vi "Fit to Decoration.vi"(8 "error in":errorcluster, 10 "Border":i32, 11 "Flex Subpanel in":refnum<class "Flex UI Subpanel.lvclass">) -> (0 "error out":errorcluster, 3 "Flex Subpanel out":refnum<class "Flex UI Subpanel.lvclass">)   [LabVIEW 2016, in "Flex UI Subpanel.lvclass"]
doc: "Resizes the subpanel around the largest decoration."
uses:
  Flex UI Subpanel.lvclass
  C:/VI Packages/Flex UI/Flex UI (Parent)/Flex UI.lvclass
  Flex UI (Parent)/Flex UI.lvclass/Flex UI.ctl
  <vilib>/Utility/miscctls.llb/LVPointTypeDef.ctl
  Flex UI Subpanel.lvclass/Flex UI Subpanel.ctl
  Flex UI (Parent)/Flex UI.lvclass
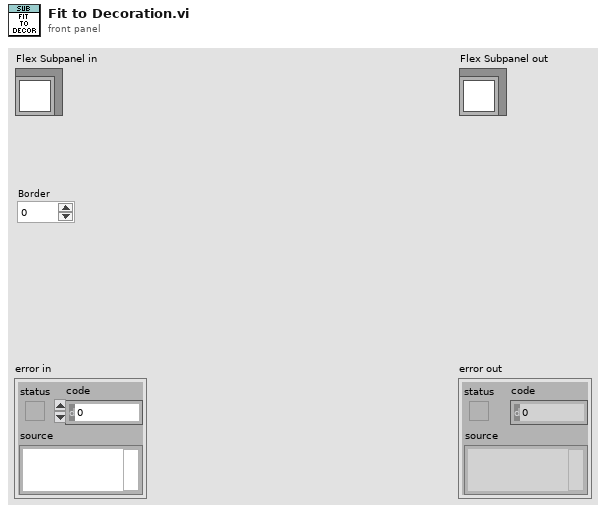
[diagram p1: front panel]
types:
  T1 = typedef "LVPointTypeDef.ctl" = cluster{"Horizontal":i16, "Vertical":i16}
  T2 = typedef "LVBoundsTypeDef.ctl" = cluster{"Width":u32, "Height":u32}
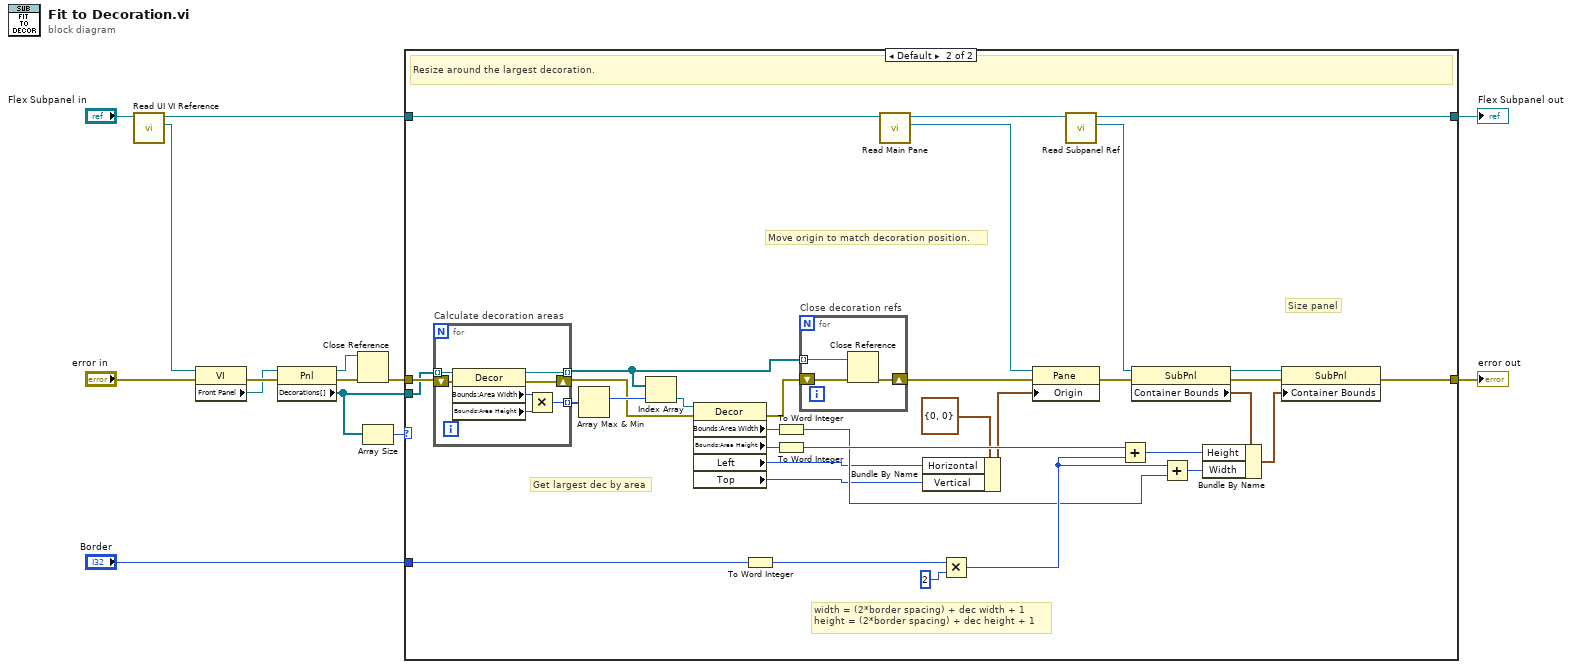
[diagram p0: block diagram]
diagram:
  n1 = call "Read UI VI Reference.vi"("Flex UI in"="Flex Subpanel in") -> ("UI VI Reference"=w8:refnum<vi>, "Flex UI out"=w11:refnum<class "Flex UI Subpanel.lvclass">)  [unwired: 9 in]
  n2 = property on="Property Node" class="VI"(reference=w8, error in="error in") -> (error out=w6:errorcluster, "Front Panel"=w4:refnum<vi>)  [unwired: 1 out]
  n3 = property on="Property Node" class="Pnl"(reference=w4, error in=w6) -> (reference out=w10:refnum<vi>, error out=w9:errorcluster, "Decorations[]"=w2:refnum<vi>[])
  n4 = Close Reference(reference=w10, error in (no error)=w9) -> (error out=w5:errorcluster)
  n5 = Array Size(array=w2) -> (size(s)=w3:i32)
  n6 = case shown="Default" w3 {
    tunnel: w5 -> [w16 w30]
    tunnel: [w16 w29] -> w14
    tunnel: [w15 w25] -> w13
    tunnel: w11 -> [w15 w28]
    tunnel: w2 -> [_ w27]
    tunnel: "Border" -> [_ w26]
    frame 0 {
      # "If no decorations are found, do nothing."
    }
    frame Default {
      # "Move origin to match decoration position."
      # "width = (2*border spacing) + dec width + 1\nheight = (2*border spacing) + dec height + 1"
      # "Size panel"
      # "Get largest dec by area"
      # "Resize around the largest decoration."
      n7 = for "Calculate decoration areas" {
        tunnel: [w55] -> w44 mode=indexing
        shift-right: [w53] -> w40
        shift-left: w30 -> [w54]
        tunnel: [w52] -> w42 mode=indexing
        tunnel: w27 -> [w51] mode=indexing
        n8 = property on="Calculate areas" class="Decor"(reference=w51, error in=w54) -> (reference out=w52:refnum<vi>, error out=w53:errorcluster, "Bounds:Area Width"=w57:u32, "Bounds:Area Height"=w56:u32)
        n9 = Multiply(x=w57, y=w56) -> (x*y=w55:u32)
      }
      n10 = Array Max & Min(array=w44) -> (max index (indices)=w43:i32)  [unwired: 3 out]
      n11 = Index Array(array=w42, index=w43) -> (element=w41:refnum<vi>)
      n12 = property class="Decor"(reference=w41, error in=w40) -> (error out=w39:errorcluster, "Bounds:Area Width"=w47:u32, "Bounds:Area Height"=w46:u32, "Left"=w18:i32, "Top"=w17:i32)  [unwired: 1 out]
      n13 = To Word Integer(number=w26) -> (16bit integer=w34:i16)
      n14 = To Word Integer(number=w47) -> (16bit integer=w32:i16)
      n15 = To Word Integer(number=w46) -> (16bit integer=w33:i16)
      n16 = for "Close decoration refs" {
        tunnel: w42 -> [w60] mode=indexing
        shift-right: [w58] -> w37
        shift-left: w39 -> [w59]
        n17 = Close Reference(reference=w60, error in (no error)=w59) -> (error out=w58:errorcluster)
      }
      n18 = call "Read Main Pane.vi"("Flex UI in"=w28) -> ("Main Pane"=w21:refnum<vi>, "Flex UI out"=w23:refnum<class "Flex UI Subpanel.lvclass">)  [unwired: 9 in]
      n19 = Bundle By Name(cluster=T1 {"Horizontal"=0, "Vertical"=0} ("Origin"), "Horizontal"=w18, "Vertical"=w17) -> (w19:T1)
      n20 = Multiply(x=w34, y=i16 2) -> (x*y=w35:i16)
      n21 = property class="Pane"(reference=w21, error in=w37, "Origin"=w19) -> (error out=w22:errorcluster)  [unwired: 1 out]
      n22 = call "Read Subpanel Ref.vi"("Flex Subpanel in"=w23) -> ("Subpanel Ref"=w24:refnum<vi>, "Flex Subpanel out"=w25:refnum<class "Flex UI Subpanel.lvclass">)  [unwired: 9 in]
      n23 = Add(x=w33, y=w35) -> (x+y=w31:i16)
      n24 = property on="Property Node" class="SubPnl"(reference=w24, error in=w22) -> (reference out=w50:refnum<vi>, error out=w36:errorcluster, "Container Bounds"=w45:T2)
      n25 = Add(x=w35, y=w32) -> (x+y=w49:i16)
      n26 = Bundle By Name(cluster=w45, "Height"=w31, "Width"=w49) -> (w48:T2)
      n27 = property on="Property Node" class="SubPnl"(reference=w50, error in=w36, "Container Bounds"=w48) -> (error out=w29:errorcluster)  [unwired: 1 out]
    }
  }
  "error out" <- w14
  "Flex Subpanel out" <- w13
